vi "Read IR Temperatures.vi"(8 "error in (no error)":errorcluster, 10 "Units":T1, 11 "Process Settings in":refnum<class "Process Settings.lvclass">) -> (0 "error out":errorcluster, 2 "Temp Cluster":T2, 3 "Process Settings out":refnum<class "Process Settings.lvclass">)   [LabVIEW 2017, in "Expansion.lvclass"]
uses:
  Expansion.lvclass
  Process Settings/Process Settings.lvclass
  Type Defs/IR Temperatures.ctl
  Process Settings/Type Defs/Units.ctl
  Hardware Settings/Type Defs/Hardware Types.ctl
  Process Settings/Process Settings.lvclass/Process Settings.ctl
  Process Settings/Accessors/Read Hardware Settings.vi
  Hardware Settings/Hardware Settings.lvclass
  Hardware Settings/Hardware Types/Generic/Generic Hardware.lvclass
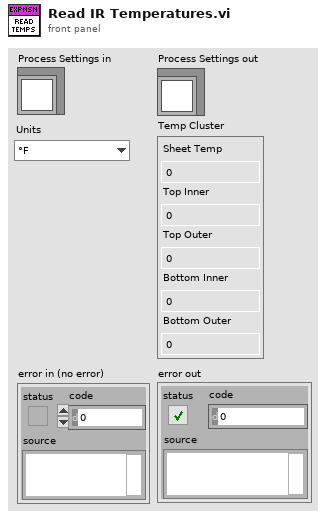
[diagram p1: front panel]
types:
  T1 = typedef "Process Settings.lvclass/Units.ctl" = enum16{"°F", "°C", "Seconds", "Minutes", "PSIA"}
  T2 = typedef "Expansion.lvclass/IR Temperatures.ctl" = cluster{"Sheet Temp":dbl, "Top Inner":dbl, "Top Outer":dbl, "Bottom Inner":dbl, "Bottom Outer":dbl}
  T3 = typedef "Hardware Settings.lvclass/Hardware Types.ctl" = enum16{"Tank Chamber Pressure and Temperature", "Tank Valve Controls", "Motor On/Off and Direction Control", "Limit Switches", "IR Temperature", "Pneumatic Cylinder Actuation", "Expansion Temperature Setpoint"}
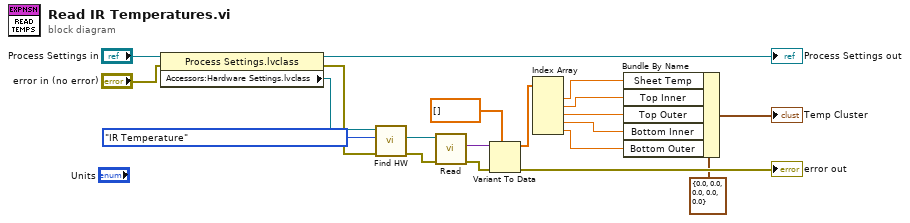
[diagram p0: block diagram]
diagram:
  n1 = property class="Process Settings.lvclass"(reference="Process Settings in", error in="error in (no error)") -> (reference out=→"Process Settings out":refnum<class "Process Settings.lvclass">, error out=w1:errorcluster, "Accessors:Hardware Settings.lvclass"=w4:refnum<class "Hardware Settings.lvclass">)
  n2 = call "Find HW.vi"("error in (no error)"=w1, "HW Item"=Hardware_Types."IR Temperature", "Hardware Settings in"=w4) -> ("error out"=w18:errorcluster, "Selected Hardware Out"=w15:refnum<class "Generic Hardware.lvclass">)  [unwired: 6 in, 1 out]
  n3 = call-dynamic "Read.vi"("error in (no error)"=w18, "Generic Hardware in"=w15) -> ("error out"=w19:errorcluster, "Output"=w16:variant)  [unwired: 7 in, 1 out]
  n4 = Variant To Data(error in=w19, type=dbl[] [], Variant=w16) -> (data=w17:dbl[], error out=→"error out":errorcluster)
  n5 = Index Array(array=w17) -> (element #1=w11:dbl, element #2=w10:dbl, element #3=w9:dbl, element #4=w7:dbl, element #5=w6:dbl)  [unwired: 5 in]
  n6 = Bundle By Name(cluster=T2 {"Sheet Temp"=0.0, "Top Inner"=0.0, "Top Outer"=0.0, "Bottom Inner"=0.0, "Bottom Outer"=0.0} ("System Cluster"), "Sheet Temp"=w11, "Top Inner"=w10, "Top Outer"=w9, "Bottom Inner"=w7, "Bottom Outer"=w6) -> (→"Temp Cluster":T2)
